vi "TcA06-002_DestroyedReferenceErrorHandling.vi"(1 "Input buffer":T3="1", 3 "Invocation info":T2, 5 "error in (no error)":errorcluster, 6 "Add log to result?":bool) -> (16 "Test Data":T1 {"Numeric Measurement" format="%.2f"}, 19 "error out":errorcluster)   [LabVIEW 2009]
doc: "Test case template."
uses:
  Shared/Support_InputBuffer.ctl
  Shared/Support_InvocationInfo.ctl
  Shared/Support_TestData.ctl
  TestClasses/G#SubSubClass1_class/G#SubSubClass1.lvclass
  TestClasses/G#BaseClass1_class/G#BaseClass1.lvclass
  TestClasses/G#SubClass1_class/G#SubClass1.lvclass
  <vilib>/addons/_AddQ/G#Object/G#Object.lvclass
panel:
  in  "Test name":string="TcA06-002 Destroyed reference error handling"
  out "Test result":bool
  out "Result":string
  # "Verify that if a reference that has been destroyed will generate\nan error code 1 if used by a method."
  # "Sub test case"
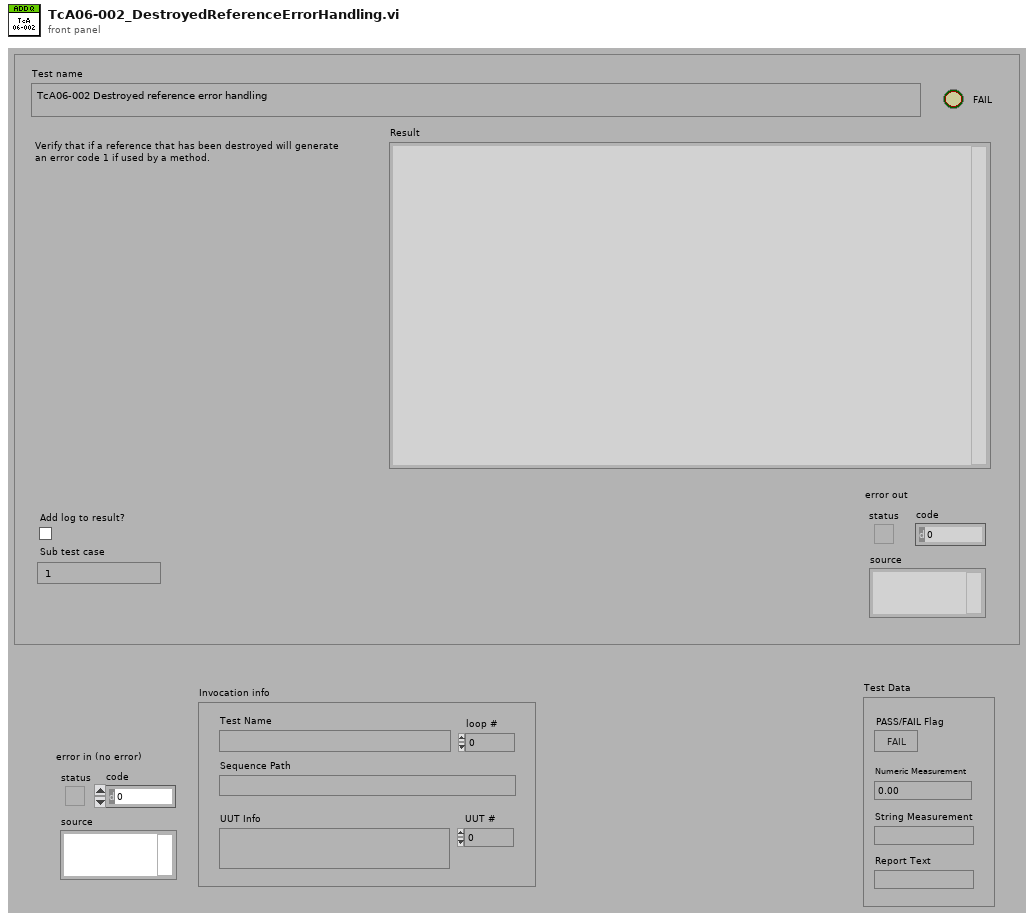
[diagram p1: front panel]
types:
  T1 = typedef "Support_TestData.ctl" = cluster{"PASS/FAIL Flag":bool, "Numeric Measurement":dbl, "String Measurement":string, "Report Text":string}
  T2 = typedef "Support_InvocationInfo.ctl" = cluster{"UUT #":i32, "loop #":i32, "UUT Info":string, "Test Name":string, "Sequence Path":path}
  T3 = typedef "Support_InputBuffer.ctl" = string
  T4 = typedef "Support_ResultType.ctl" = cluster{"Pass":bool, "Comment":string, "MeasurementValue":dbl}
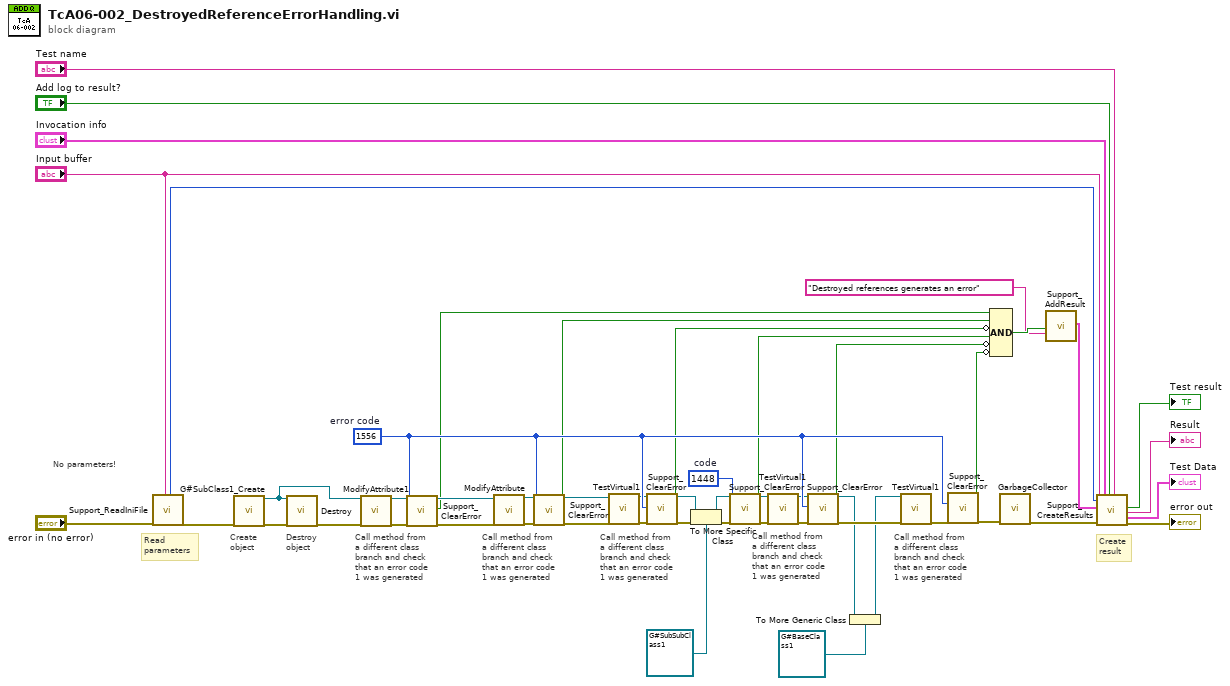
[diagram p0: block diagram]
diagram:
  w2 = 1448  # code
  w25 = 1556  # error code
  # "Destroy\nobject"
  # "No parameters!"
  # "Call method from\na different class\nbranch and check\nthat an error code\n1 was generated"
  # "Call method from\na different class\nbranch and check\nthat an error code\n1 was generated"
  # "Call method from\na different class\nbranch and check\nthat an error code\n1 was generated"
  # "Call method from\na different class\nbranch and check\nthat an error code\n1 was generated"
  # "Call method from\na different class\nbranch and check\nthat an error code\n1 was generated"
  # "Create\nobject"
  # "Create\nresult"
  # "Read\nparameters"
  n1 = call "Support_ReadIniFile.vi"("error in (no error)"="error in (no error)", "Sub test case"="Input buffer") -> ("Timer start"=w36:u32, "error out"=w32:errorcluster)  [unwired: 10 in, 6 out]
  n2 = call "G#SubClass1_Create.vi"("error in (no error)"=w32) -> ("reference out"=w12:refnum<class "G#SubClass1.lvclass">, "error out"=w14:errorcluster)  [unwired: 16 in, 1 out]
  n3 = call-dynamic "Destroy.vi"("reference in"=w12, "error in (no error)"=w14) -> ("error out"=w13:errorcluster)  [unwired: 16 in, 1 out]
  n4 = call-dynamic "ModifyAttribute1.vi"("reference in"=w12, "error in (no error)"=w13) -> ("reference out"=w34:refnum<class "G#SubClass1.lvclass">, "error out"=w31:errorcluster)  [unwired: 16 in]
  n5 = call "Support_ClearError.vi"("code"=w25, "error in (no error)"=w31) -> ("Cleared?"=w23:bool, "error out"=w30:errorcluster)  [unwired: 16 in]
  n6 = call-dynamic "ModifyAttribute.vi"("reference in"=w34, "error in (no error)"=w30) -> ("reference out"=w33:refnum<class "G#SubClass1.lvclass">, "error out"=w29:errorcluster)  [unwired: 16 in]
  n7 = call "Support_ClearError.vi"("code"=w25, "error in (no error)"=w29) -> ("Cleared?"=w22:bool, "error out"=w28:errorcluster)  [unwired: 16 in]
  n8 = call-dynamic "TestVirtual1.vi"("reference in"=w33, "error in (no error)"=w28) -> ("reference out"=w10:refnum<class "G#SubClass1.lvclass">, "error out"=w27:errorcluster)  [unwired: 15 in, 1 out]
  n9 = call "Support_ClearError.vi"("code"=w25, "error in (no error)"=w27) -> ("Cleared?"=w21:bool, "error out"=w5:errorcluster)  [unwired: 16 in]
  n10 = To More Specific Class(target class=refnum<class "G#SubSubClass1.lvclass"> refnum ("G#SubSubClass1.lvclass"), reference=w10, error in=w5) -> (specific class reference=w9:refnum<class "G#SubSubClass1.lvclass">, error out=w3:errorcluster)
  n11 = call "Support_ClearError.vi"("code"=w2, "error in (no error)"=w3) -> ("Cleared?"=w1:bool, "error out"=w4:errorcluster)  [unwired: 16 in]
  n12 = call-dynamic "TestVirtual1.vi"("reference in"=w9, "error in (no error)"=w4) -> ("reference out"=w7:refnum<class "G#SubSubClass1.lvclass">, "error out"=w26:errorcluster)  [unwired: 15 in, 1 out]
  n13 = call "Support_ClearError.vi"("code"=w25, "error in (no error)"=w26) -> ("Cleared?"=w20:bool, "error out"=w17:errorcluster)  [unwired: 16 in]
  n14 = To More Generic Class(target class=refnum<class "G#BaseClass1.lvclass"> refnum ("G#BaseClass1.lvclass"), reference=w7) -> (generic class reference=w6:refnum<class "G#BaseClass1.lvclass">)
  n15 = call-dynamic "TestVirtual1.vi"("reference in"=w6, "error in (no error)"=w17) -> ("error out"=w16:errorcluster)  [unwired: 15 in, 2 out]
  n16 = call "Support_ClearError.vi"("code"=w25, "error in (no error)"=w16) -> ("Cleared?"=w19:bool, "error out"=w15:errorcluster)  [unwired: 16 in]
  n17 = Compound Arithmetic op=AND(w23, w22, invert w21, w1, invert w20, invert w19) -> (w24:bool)
  n18 = call <vilib>:"GarbageCollector.vi"("error in (no error)"=w15) -> ("error out"=w35:errorcluster)  [unwired: 16 in, 2 out]
  n19 = call "Support_AddResult.vi"("Pass"=w24, "Comment"="Destroyed references generates an error") -> ("Results out"=w39:T4[])  [unwired: 17 in]
  n20 = call "Support_CreateResults.vi"("Sub test case"="Input buffer", "Timer start"=w36, "Results"=w39, "error in (no error)"=w35, "Invocation info"="Invocation info", "Add log to result?"="Add log to result?", "Test name"="Test name") -> ("Pass/fail flag"=→"Test result":bool, "Result"=→"Result":string, "Test Data"=→"Test Data":T1, "error out"=→"error out":errorcluster)  [unwired: 9 in]
